vi "Path Resolve.vi"(7 "additional search path":path, 8 "Error In":errorcluster, 10 "create?":bool, 11 "absolute or relative path":path) -> (0 "Error Out":errorcluster, 3 "resolved path":path)   [LabVIEW 2015]
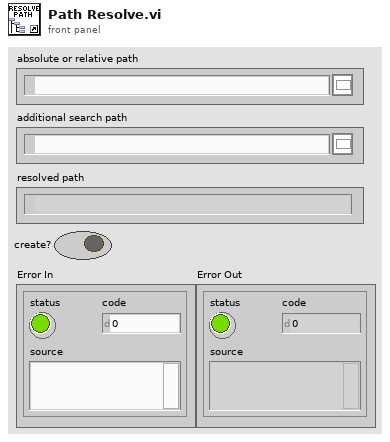
[diagram p1: front panel]
types:
  T1 = enum16{"open", "replace", "create", "open or create", "replace or create", "replace or create with confirmation"}
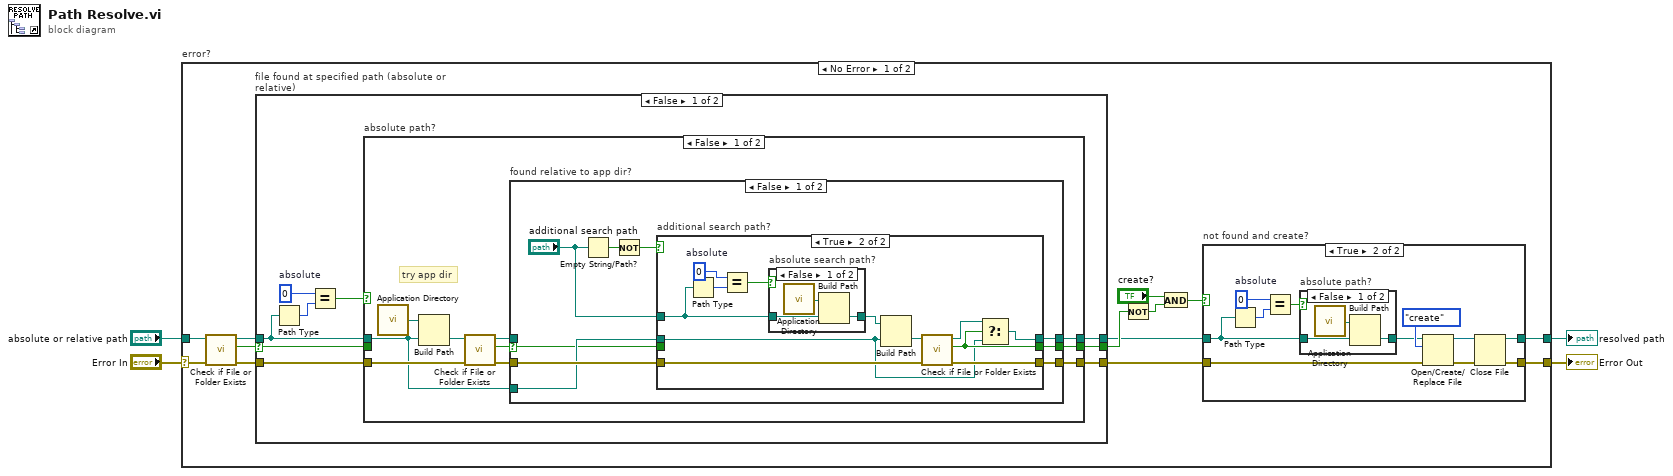
[diagram p0: block diagram]
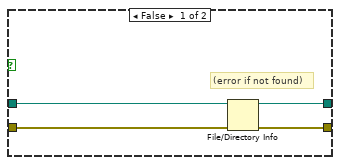
[diagram p2: hidden frame]
diagram:
  n1 = case "error?" shown="No Error" "Error In" {
    selector: "Error In" -> [w16 w93]
    tunnel: "absolute or relative path" -> [w17 w94]
    tunnel: [w5 w93] -> w3
    tunnel: [w6 w94] -> w2
    frame No Error {
      n2 = call <vilib>:"Check if File or Folder Exists.vi"("error in (no error)"=w16, "path"=w17) -> ("error out"=w14:errorcluster, "file or folder exists?"=w13:bool, "dup path"=w15:path)  [unwired: 7 in]
      n3 = case "file found at specified path (absolute or relative)" shown="False" w13 {
        selector: w13 -> [w41 w90]
        tunnel: [w45 w91] -> w7
        tunnel: [w44 w92] -> w8
        tunnel: w15 -> [w40 w92]
        tunnel: w14 -> [w43 w91]
        tunnel: [w42 w90] -> w9
        frame False {
          w38 = i16 0  # absolute
          n4 = Path Type(1:w40) -> (0:w39:i16)
          n5 = Equal?(x=w38, y=w39) -> (x = y?=w37:bool)
          n6 = case "absolute path?" shown="False" w37 {
            tunnel: w40 -> [w46 w88]
            tunnel: w43 -> [w55 w89]
            tunnel: [w49 w88] -> w44
            tunnel: [w48 w89] -> w45
            tunnel: [w47 w87] -> w42
            tunnel: w41 -> [_ w87]
            frame False {
              # "try app dir"
              n7 = call <vilib>:"Application Directory.vi"() -> ("Application Directory"=w54:path)
              n8 = Build Path(base path=w54, name or relative path=w46) -> (appended path=w53:path)
              n9 = call <vilib>:"Check if File or Folder Exists.vi"("error in (no error)"=w55, "path"=w53) -> ("error out"=w50:errorcluster, "file or folder exists?"=w52:bool, "dup path"=w51:path)  [unwired: 7 in]
              n10 = case "found relative to app dir?" shown="False" w52 {
                selector: w52 -> [w56 w84]
                tunnel: w51 -> [_ w86]
                tunnel: w50 -> [w58 w85]
                tunnel: [w61 w86] -> w49
                tunnel: [w59 w85] -> w48
                tunnel: [w60 w84] -> w47
                tunnel: w46 -> [w57 _]
                frame False {
                  n11 = Empty String/Path?(string/path="additional search path") -> (empty?=w64:bool)
                  n12 = Not(x=w64) -> (.not. x?=w63:bool)
                  n13 = case "additional search path?" shown="True" w63 {
                    tunnel: "additional search path" -> [_ w76]
                    tunnel: w57 -> [w67 w68]
                    tunnel: [w67 w69] -> w61
                    tunnel: [w66 w70] -> w60
                    tunnel: [w65 w74] -> w59
                    tunnel: w58 -> [w65 w73]
                    tunnel: w56 -> [w66 _]
                    frame False {
                    }
                    frame True {
                      w78 = i16 0  # absolute
                      n14 = Path Type(1:w76) -> (0:w79:i16)
                      n15 = Equal?(x=w78, y=w79) -> (x = y?=w77:bool)
                      n16 = case "absolute search path?" shown="False" w77 {
                        tunnel: [w81 w83] -> w75
                        tunnel: w76 -> [w80 w83]
                        frame False {
                          n17 = call <vilib>:"Application Directory.vi"() -> ("Application Directory"=w82:path)
                          n18 = Build Path(base path=w82, name or relative path=w80) -> (appended path=w81:path)
                        }
                        frame True {
                        }
                      }
                      n19 = Build Path(base path=w75, name or relative path=w68) -> (appended path=w72:path)
                      n20 = call <vilib>:"Check if File or Folder Exists.vi"("error in (no error)"=w73, "path"=w72) -> ("error out"=w74:errorcluster, "file or folder exists?"=w70:bool, "dup path"=w71:path)  [unwired: 7 in]
                      n21 = Select(t=w71, s=w70, f=w68) -> (s? t:f=w69:path)
                    }
                  }
                }
                frame True {
                }
              }
            }
            frame True {
            }
          }
        }
        frame True {
        }
      }
      n22 = Not(x=w9) -> (.not. x?=w12:bool)
      n23 = And(x="create?", y=w12) -> (x .and. y?=w11:bool)
      n24 = case "not found and create?" shown="True" w11 {
        tunnel: w7 -> [w21 w32]
        tunnel: w8 -> [w19 w23]
        tunnel: [w18 w28] -> w6
        tunnel: [w20 w27] -> w5
        frame False {
          # "(error if not found)"
          n25 = File/Directory Info(path=w19, error in=w21) -> (path out=w18:path, error out=w20:errorcluster)  [unwired: 5 out]
        }
        frame True {
          w25 = i16 0  # absolute
          n26 = Path Type(1:w23) -> (0:w26:i16)
          n27 = Equal?(x=w25, y=w26) -> (x = y?=w24:bool)
          n28 = case "absolute path?" shown="False" w24 {
            tunnel: [w34 w36] -> w22
            tunnel: w23 -> [w33 w36]
            frame False {
              n29 = call <vilib>:"Application Directory.vi"() -> ("Application Directory"=w35:path)
              n30 = Build Path(base path=w35, name or relative path=w33) -> (appended path=w34:path)
            }
            frame True {
            }
          }
          n31 = Open/Create/Replace File(file path (use dialog)=w22, error in=w32, operation (0:open)=T1."create") -> (refnum out=w29:refnum<file>, error out=w30:errorcluster)  [unwired: 3 in, 1 out]
          n32 = Close File(refnum=w29, error in=w30) -> (path=w28:path, error out=w27:errorcluster)
        }
      }
    }
    frame Error {
    }
  }
  "resolved path" <- w2
  "Error Out" <- w3
